vi "2D_tip-generation.vi"(5 "Angle":dbl=20.0 min=1.0 max=89.0 format="%.2f", 6 "Radius":dbl=10.0 min=-0.0 max=1000.0 format="%.2f", 7 "Tip height":dbl=10.0 format="%#_13g", 8 "Position Y":i32=500, 9 "Position X":i32=500, 10 "Pixels Y":i32=500, 11 "Pixels X":i32=500) -> (1 "Tip section":dbl[](graph)=[0.0, 0.0, 0.0, 0.0, 0.0, 0.0, 0.0, 0.0, 0.0, 0.0, 0.0, 0.0, 0.0, 0.0, 0.0, 0.0, 0.0, 0.0, 0.0, 0.0, 0.0, 0.0, 0.0, 0.0, 0.0, 0.0, 0.0, 0.0, 0.0, 0.0, 0.0, 0.0, 0.0, 0.0, 0.0, 0.0, 0.0, 0.0, 0.0, 0.0, 0.0, 0.0, 0.0, 0.0, 0.0, 0.0, 0.0, 0.0, 0.0, 0.0, 0.0, 0.0, 0.0, 0.0, 0.0, 0.0, 0.0, 0.0, 0.0, 0.0, 0.0, 0.0, 0.0, 0.0, 0.0, 0.0, 0.0, 0.0, 0.0, 0.0, 0.0, 0.0, 0.0, 0.0, 0.0, 0.0, 0.0, 0.0, 0.0, 0.0, 0.0, 0.0, 0.0, 0.0, 0.0, 0.0, 0.0, 0.0, 0.0, 0.0, 0.0, 0.0, 0.0, 0.0, 0.0, 0.0, 0.0, 0.0, 0.0, 0.0, 0.0, 0.0, 0.0, 0.0, 0.0, 0.0, 0.0, 0.0, 0.0, 0.0, 0.0, 0.0, 0.0, 0.0, 0.0, 0.0, 0.0, 0.0, 0.0, 0.0, 0.0, 0.0, 0.0, 0.0, 0.0, 0.0, 0.0, 0.0, 0.0, 0.0, 0.0, 0.0, 0.0, 0.0, 0.0, 0.0, 0.0, 0.0, 0.0, 0.0, 0.0, 0.0, 0.0, 0.0, 0.0, 0.0, 0.0, 0.0, 0.0, 0.0, 0.0, 0.0, 0.0, 0.0, 0.0, 0.0, 0.0, 0.0, 0.0, 0.0, 0.0, 0.0, 0.0, 0.0, 0.0, 0.0, 0.0, 0.0, 0.0, 0.0, 0.0, 0.0, 0.0, 0.0, 0.0, 0.0, 0.0, 0.0, 0.0, 0.0, 0.0, 0.0, 0.0, 0.0, 0.0, 0.0, 0.0, 0.0, 0.0, 0.0, 0.0, 0.0, 0.0, 0.0, 0.0, 0.0, 0.0, 0.0, 0.0, 0.0, 0.0, 0.0, 0.0, 0.0, 0.0, 0.0, 0.0, 0.0, 0.0, 0.0, 0.0, 0.0, 0.0, 0.0, 0.0, 0.0, 0.0, 0.0, 0.0, 0.0, 0.0, 0.0, 0.0, 0.0, 0.0, 0.0, 0.0, 0.0, 0.0, 0.0, 0.0, 0.0, 0.0, 0.0, 0.0, 0.0, 0.0, 0.0, 0.0, 1.7632698070846526, 4.358898943540674, 6.0, 7.14142842854285, 8.0, 8.660254037844387, 9.16515138991168, 9.539392014169456, 9.797958971132712, 9.9498743710662, 10.0, 9.9498743710662, 10.0, 9.9498743710662, 9.797958971132712, 9.539392014169456, 9.16515138991168, 8.660254037844387, 8.0, 7.14142842854285, 6.0, 4.358898943540674, 1.7632698070846526, 0.0, 0.0, 0.0, 0.0, 0.0, 0.0, 0.0, 0.0, 0.0, 0.0, 0.0, 0.0, 0.0, 0.0, 0.0, 0.0, 0.0, 0.0, 0.0, 0.0, 0.0, 0.0, 0.0, 0.0, 0.0, 0.0, 0.0, 0.0, 0.0, 0.0, 0.0, 0.0, 0.0, 0.0, 0.0, 0.0, 0.0, 0.0, 0.0, 0.0, 0.0, 0.0, 0.0, 0.0, 0.0, 0.0, 0.0, 0.0, 0.0, 0.0, 0.0, 0.0, 0.0, 0.0, 0.0, 0.0, 0.0, 0.0, 0.0, 0.0, 0.0, 0.0, 0.0, 0.0, 0.0, 0.0, 0.0, 0.0, 0.0, 0.0, 0.0, 0.0, 0.0, 0.0, 0.0, 0.0, 0.0, 0.0, 0.0, 0.0, 0.0, 0.0, 0.0, 0.0, 0.0, 0.0, 0.0, 0.0, 0.0, 0.0, 0.0, 0.0, 0.0, 0.0, 0.0, 0.0, 0.0, 0.0, 0.0, 0.0, 0.0, 0.0, 0.0, 0.0, 0.0, 0.0, 0.0, 0.0, 0.0, 0.0, 0.0, 0.0, 0.0, 0.0, 0.0, 0.0, 0.0, 0.0, 0.0, 0.0, 0.0, 0.0, 0.0, 0.0, 0.0, 0.0, 0.0, 0.0, 0.0, 0.0, 0.0, 0.0, 0.0, 0.0, 0.0, 0.0, 0.0, 0.0, 0.0, 0.0, 0.0, 0.0, 0.0, 0.0, 0.0, 0.0, 0.0, 0.0, 0.0, 0.0, 0.0, 0.0, 0.0, 0.0, 0.0, 0.0, 0.0, 0.0, 0.0, 0.0, 0.0, 0.0, 0.0, 0.0, 0.0, 0.0, 0.0, 0.0, 0.0, 0.0, 0.0, 0.0, 0.0, 0.0, 0.0, 0.0, 0.0, 0.0, 0.0, 0.0, 0.0, 0.0, 0.0, 0.0, 0.0, 0.0, 0.0, 0.0, 0.0, 0.0, 0.0, 0.0, 0.0, 0.0, 0.0, 0.0, 0.0, 0.0, 0.0, 0.0, 0.0, 0.0, 0.0, 0.0, 0.0, 0.0, 0.0, 0.0, 0.0, 0.0, 0.0, 0.0, 0.0, 0.0, 0.0, 0.0, 0.0, 0.0, 0.0, 0.0, 0.0, 0.0, 0.0, 0.0, 0.0, 0.0, 0.0, 0.0, 0.0, 0.0, 0.0, 0.0, 0.0, 0.0, 0.0, 0.0, 0.0, 0.0], 2 "2D Tip":dbl[][](graph))   [LabVIEW 2017]
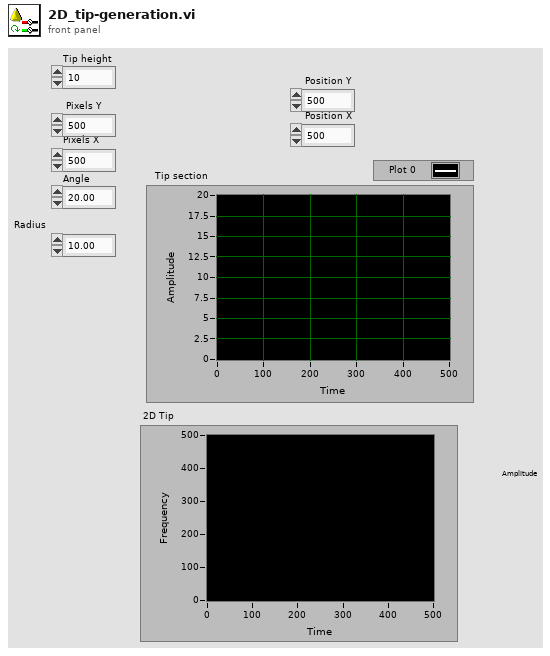
[diagram p1: front panel]
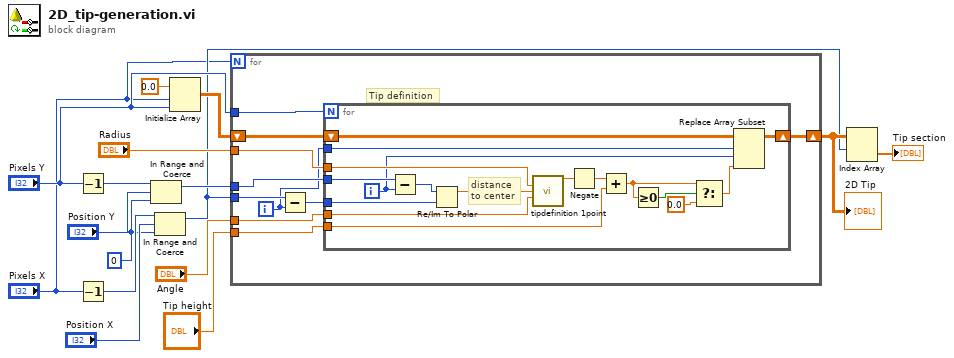
[diagram p0: block diagram]
diagram:
  w1 = 0 ("lower limit")
  n1 = Decrement(x="Pixels Y") -> (x-1=w6:i32)
  n2 = Decrement(x="Pixels X") -> (x-1=w5:i32)
  n3 = In Range and Coerce(upper limit=w6, x="Position Y", lower limit=w1) -> (coerced(x)=w9:i32)  [unwired: 1 out]
  n4 = In Range and Coerce(upper limit=w5, x="Position X", lower limit=w1) -> (coerced(x)=w3:i32)  [unwired: 1 out]
  n5 = Initialize Array(0.0 ("element"), "Pixels X", "Pixels Y") -> (w13:dbl[][])
  n6 = for {
    N: "Pixels X" -> [_]
    tunnel: "Pixels Y" -> [w26]
    tunnel: w3 -> [w24]
    tunnel: w9 -> [w25]
    tunnel: "Radius" -> [w23]
    tunnel: "Angle" -> [w22]
    shift-right: [w20] -> w11
    shift-left: w13 -> [w21]
    tunnel: "Tip height" -> [w17]
    i -> [w19]
    # "Tip definition"
    n7 = Subtract(x=w24, y=w19) -> (x-y=w18:i32)
    n8 = for {
      N: w26 -> [_]
      tunnel: w25 -> [w43]
      tunnel: w23 -> [w42]
      tunnel: w22 -> [w41]
      shift-right: [w40] -> w20
      shift-left: w21 -> [w39]
      tunnel: w19 -> [w37]
      tunnel: w18 -> [w35]
      tunnel: w17 -> [w27]
      i -> [w38]
      # "distance\nto center"
      n9 = Subtract(x=w43, y=w38) -> (x-y=w36:i32)
      n10 = Re/Im To Polar(2:w35, 3:w36) -> (1:w34:dbl)  [unwired: 1 out]
      n11 = call "tipdefinition 1point.vi"("radius of curvature"=w42, "x"=w34, "tipangle"=w41) -> ("result"=w33:dbl)  [unwired: 12 in]
      n12 = Negate(x=w33) -> (-x=w32:dbl)
      n13 = Add(x=w32, y=w27) -> (x+y=w30:dbl)
      n14 = Greater Or Equal To 0?(x=w30) -> (x >= 0?=w31:bool)
      n15 = Select(t=w30, s=w31, f=0.0) -> (s? t:f=w28:dbl)
      n16 = Replace Array Subset(array=w39, new element=w28, index (row)=w37, index (col)=w38) -> (w40:dbl[][])
    }
  }
  "2D Tip" <- w11
  n17 = Index Array(array=w11, index (row)=w3) -> (element=→"Tip section":dbl[])  [unwired: 1 in]
